vi "Add subscription.vi"(8 "error in (no error)":errorcluster, 9 "pointer":i64, 10 "PV name":string, 11 "Client in":refnum<class "Client.lvclass">) -> (0 "error out":errorcluster, 3 "Client out":refnum<class "Client.lvclass">)   [LabVIEW 2020, in "Client.lvlib" / "Client.lvclass"]
uses:
  Client.lvclass
  Client.lvclass/Client.ctl
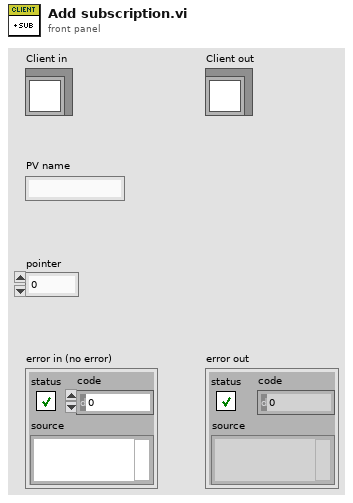
[diagram p1: front panel]
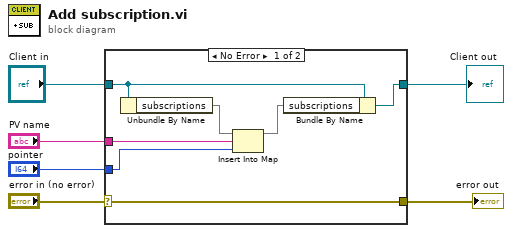
[diagram p0: block diagram]
diagram:
  n1 = case shown="No Error" "error in (no error)" {
    selector: "error in (no error)" -> [w13 w14]
    tunnel: [w13 w14] -> w5
    tunnel: [w9 w15] -> w3
    tunnel: "Client in" -> [w10 w15]
    tunnel: "PV name" -> [w8 _]
    tunnel: "pointer" -> [w7 _]
    frame No Error {
      n2 = Unbundle By Name(w10) -> ("subscriptions"=w12:map{string, i64})
      n3 = Insert Into Map(map in=w12, key=w8, value=w7) -> (map out=w11:map{string, i64})  [unwired: 2 out]
      n4 = Bundle By Name(cluster=w10, "subscriptions"=w11) -> (w9:refnum<class "Client.lvclass">)
    }
    frame Error {
    }
  }
  "error out" <- w5
  "Client out" <- w3
